vi "GetSquareWaveGenStatus.vi"(8 "error in (no error)":errorcluster) -> (0 "error out":errorcluster, 3 "function return":i16)   [LabVIEW 2013, in "HS3OverallRoutines.lvlib"]
doc: "Some instruments have a built-in square wave generator, the\nHS508 for example. This routine checks the presence of the\ngenerator.\n\nInput: -\nOutput: Return value E_NO_ERRORS | E_NO_GENERATOR | E_NO_HARDWARE\n\n\n\nshort int GetSquareWaveGenStatus ( void );"
uses:
  HS3OverallRoutines.lvlib
  hs3.dll
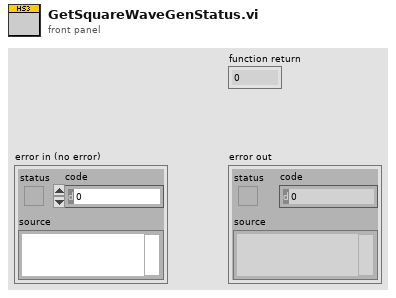
[diagram p1: front panel]
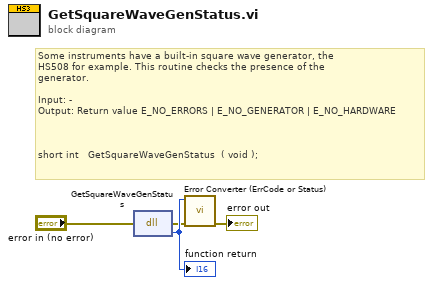
[diagram p0: block diagram]
diagram:
  # "Some instruments have a built-in square wave generator, the\nHS508 for example. This routine checks the presence of the\ngenerator.\n\nInput: -\nOutput: Return value E_NO_ERRORS | E_NO_GENERATOR | E_NO_HARDWARE\n\n\n\nshort int \t\tGetSquareWaveGenStatus\t\t( void );"
  n1 = dll-call lib="C:/Documents and Settings/admin/Pulpit/HS3 LabViewLib/HS3_WRAPPER/OverallRoutines/hs3.*" fn="GetSquareWaveGenStatus"(error in="error in (no error)") -> (error out=w2:errorcluster, w4:i16)  [unwired: 2 in, 1 out]
  "function return" <- w4
  n2 = call "Error Converter (ErrCode or Status).vi"("error in (no error)"=w2, "error code"=w4) -> ("error out"=→"error out":errorcluster)  [unwired: 9 in]
